vi "PDU Get All Outlets.vi"(8 "error in (no error)":errorcluster, 11 "Orion PDU in":refnum<class "Orion PDU.lvclass">) -> (0 "error out":errorcluster, 1 "current":dbl, 2 "States":bool[](array[boolean]), 3 "Orion PDU out":refnum<class "Orion PDU.lvclass">)   [LabVIEW 2022 SP3, in "Orion PDU.lvclass"]
uses:
  Orion PDU.lvclass
  C:/Development/rimas/RIMAS/Power Distribution/Power Distribution.lvclass
  Orion PDU.lvclass/Orion PDU.ctl
  Power Distribution.lvclass/Power Distribution.ctl
  Power Distribution.lvclass
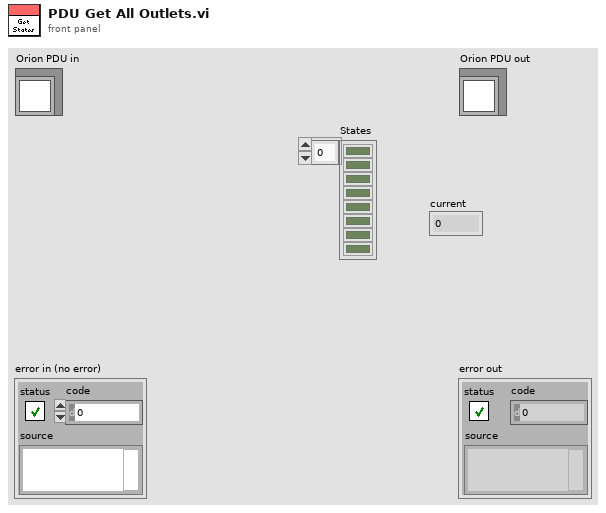
[diagram p1: front panel]
types:
  T1 = typedef "LabVIEWHTTPClient.lvlib/ClientHandle.ctl" = refnum<k1>
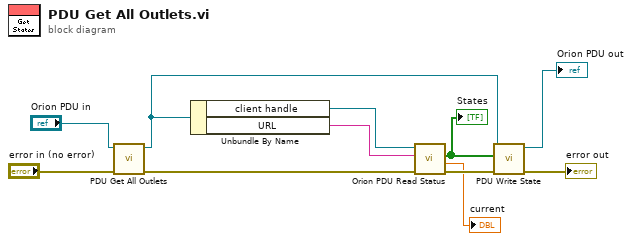
[diagram p0: block diagram]
diagram:
  n1 = call-parent "PDU Get All Outlets.vi"("error in (no error)"="error in (no error)", "Power Distribution in"="Orion PDU in") -> ("error out"=w7:errorcluster, "Power Distribution out"=w6:refnum<class "Orion PDU.lvclass">)  [unwired: 6 in, 2 out]
  n2 = Unbundle By Name(w6) -> ("client handle"=w9:T1, "URL"=w8:string)
  n3 = call "Orion PDU Read Status.vi"("error in (no error)"=w7, "Address"=w8, "client handle"=w9) -> ("error out"=w3:errorcluster, "current"=→"current":dbl, "states"=w4:bool[])  [unwired: 5 in, 1 out]
  "States" <- w4
  n4 = call "PDU Write State.vi"("error in (no error)"=w3, "State"=w4, "Power Distribution in"=w6) -> ("error out"=→"error out":errorcluster, "Power Distribution out"=→"Orion PDU out":refnum<class "Orion PDU.lvclass">)  [unwired: 7 in]
